vi "X_Y_movePID.vi"() -> ()   [LabVIEW 2023]
doc: "Shows how to move a motor to an absolute position."
panel:
  out "function name out":errorcluster
  out "element 2":dbl
  in  "Home 2":bool
  in  "HWSerialNum 2":i32=83829481
  in  "MG17Motor 2":refnum<k7>(container)
  out "element":dbl
  out "return value":dbl[](array[numeric])
  in  "HWSerialNum":i32=83828425
  in  "MG17Motor":refnum<k7>(container)
  in  "Stop":bool
  in  "Home":bool
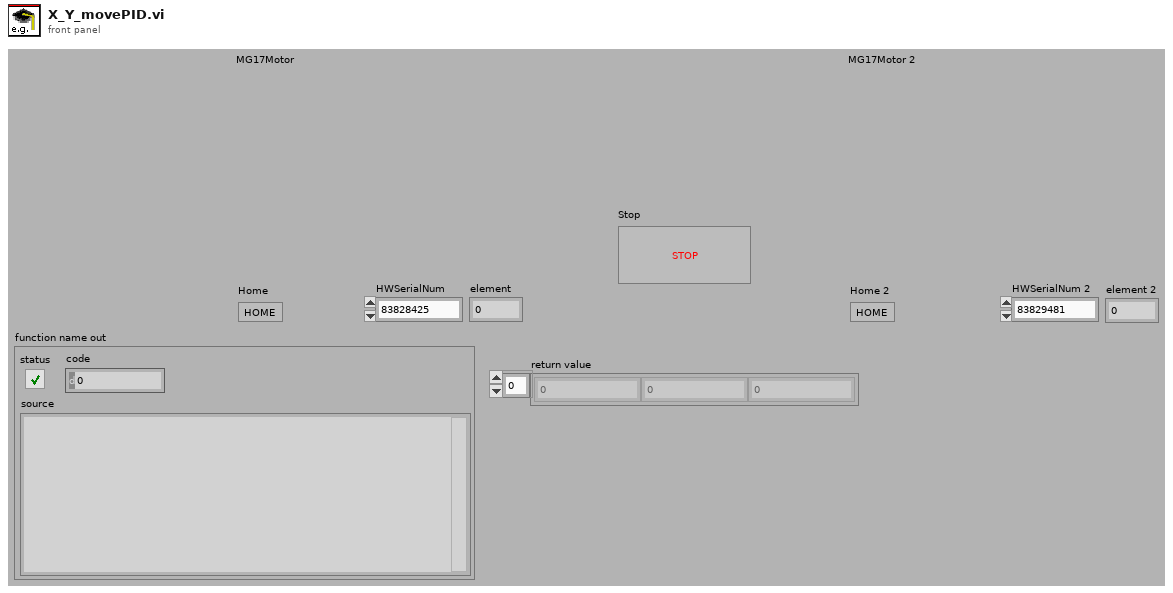
[diagram p1: front panel]
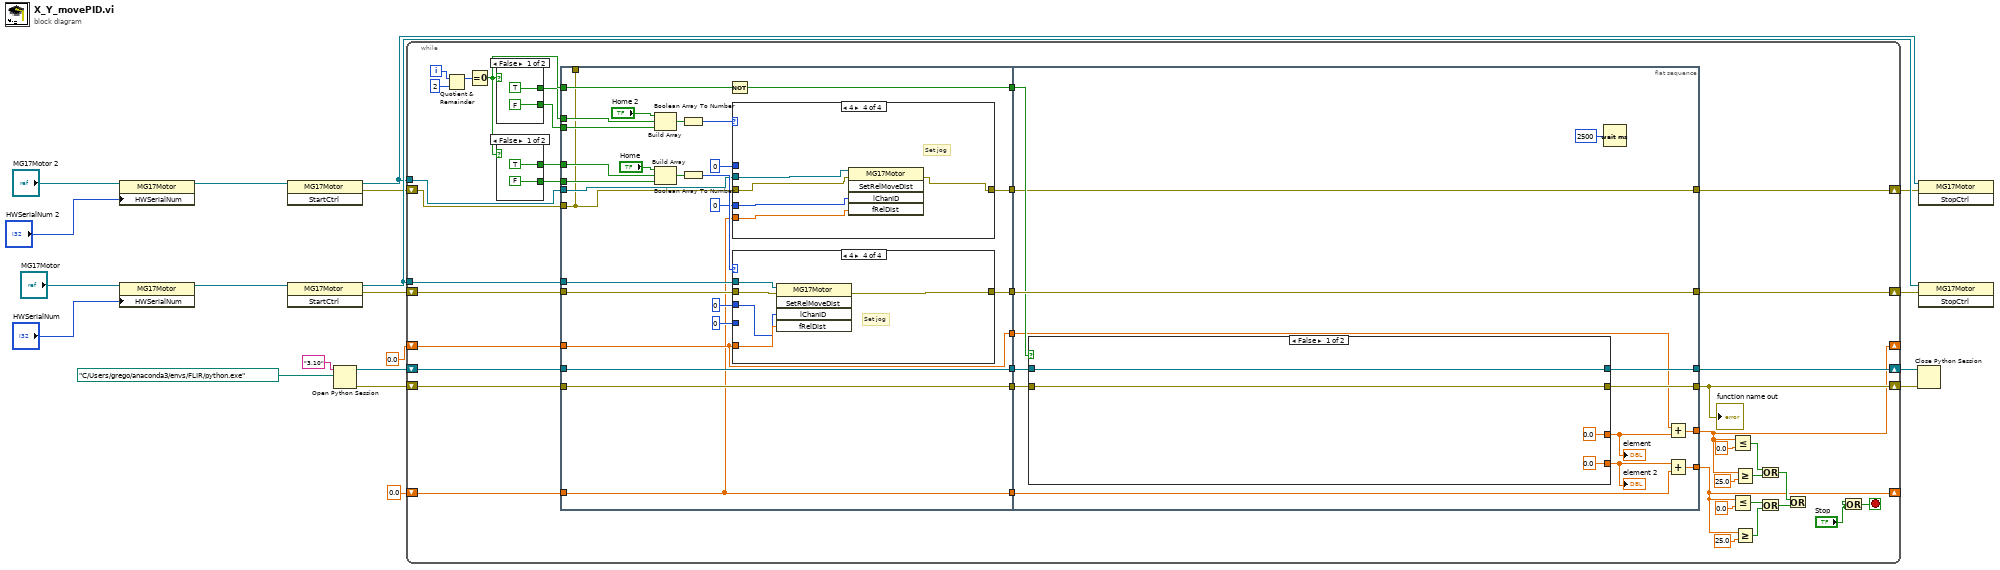
[diagram p0: block diagram]
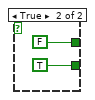
[diagram p2: hidden frame]
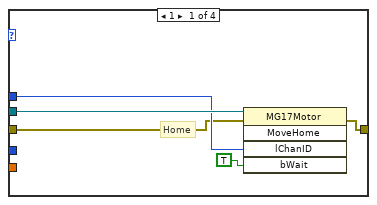
[diagram p3: hidden frame]
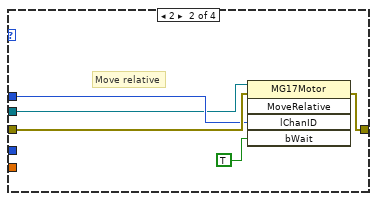
[diagram p4: hidden frame]
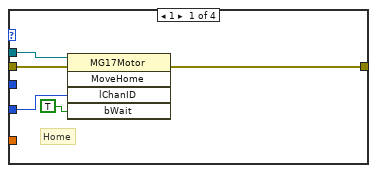
[diagram p6: hidden frame]
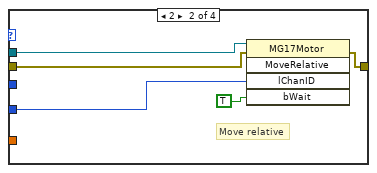
[diagram p7: hidden frame]
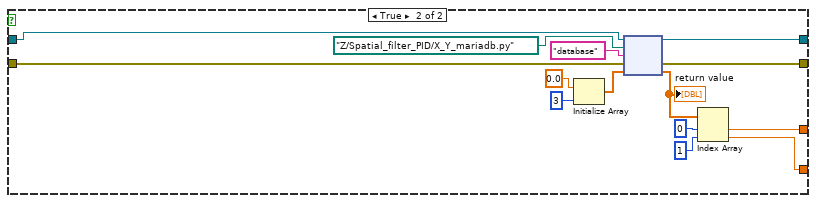
[diagram p9: hidden frame]
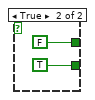
[diagram p10: hidden frame]
diagram:
  n1 = property class="MG17Motor"(reference="MG17Motor 2", "HWSerialNum"="HWSerialNum 2") -> (reference out=w8:refnum<k7>)  [unwired: 1 in, 1 out]
  n2 = property class="MG17Motor"(reference="MG17Motor", "HWSerialNum"="HWSerialNum") -> (reference out=w17:refnum<k7>)  [unwired: 1 in, 1 out]
  n3 = invoke class="MG17Motor" method="StartCtrl"(reference=w8) -> (reference out=w4:refnum<k7>, error out=w3:errorcluster)  [unwired: 2 in, 1 out]
  n4 = invoke class="MG17Motor" method="StartCtrl"(reference=w17) -> (reference out=w20:refnum<k7>, error out=w19:errorcluster)  [unwired: 2 in, 1 out]
  n5 = Open Python Session(python version="3.10" ("Python version"), python path=path "C:/Users/grego/anaconda3/envs/FLIR/python.exe" ("Python path")) -> (session out=w12:refnum<k35>, error out=w11:errorcluster)  [unwired: 1 in]
  n6 = while {
    shift-left: w19 -> [w59]
    shift-right: [w60] -> w18
    tunnel: w20 -> [w61]
    shift-right: [w42] -> _
    shift-left: 0.0 ("p") -> [w53]
    shift-right: [w50] -> w10
    shift-left: w12 -> [w47]
    shift-right: [w49] -> w9
    shift-left: w11 -> [w45]
    tunnel: w4 -> [w36]
    shift-right: [w26] -> _
    shift-left: 0.0 -> [w33]
    shift-right: [w25] -> w5
    shift-left: w3 -> [w23]
    i -> [w57]
    stop <- w24 stop-if-true
    n7 = Quotient & Remainder(x=w57, y=2) -> (x-y*floor(x/y)=w58:i32)  [unwired: 1 out]
    n8 = Equal To 0?(x=w58) -> (x = 0?=w37:bool)
    n9 = case shown="False" w37 {
      tunnel: [TRUE FALSE] -> w35
      tunnel: [FALSE TRUE] -> w34
      frame False {
      }
      frame True {
      }
    }
    n10 = case shown="False" w37 {
      tunnel: [TRUE FALSE] -> w55
      tunnel: [FALSE TRUE] -> w54
      frame False {
      }
      frame True {
      }
    }
    n11 = flat-sequence {
      tunnel: w61 -> [w90]
      tunnel: w59 -> [w87]
      tunnel: w55 -> [w70]
      tunnel: w54 -> [w69]
      tunnel: w53 -> [w79]
      tunnel: w37 -> [w83]
      tunnel: [w88] -> w52
      tunnel: [w82] -> w51
      tunnel: [w81] -> w48
      tunnel: w47 -> [w81]
      tunnel: [w80] -> w46
      tunnel: w45 -> [w80]
      tunnel: [w79] -> w44
      tunnel: w36 -> [w78]
      tunnel: [w66] -> _
      tunnel: w35 -> [w76]
      tunnel: w34 -> [w75]
      tunnel: w33 -> [w67]
      tunnel: [w68] -> w32
      tunnel: [w67] -> w31
      tunnel: w23 -> [w66]
      tunnel: [w137] -> w60
      tunnel: w52 -> [w137]
      tunnel: w51 -> [w134]
      tunnel: [w136] -> w50
      tunnel: [w135] -> w49
      tunnel: [w131] -> w42
      tunnel: w48 -> [w132]
      tunnel: w46 -> [w133]
      tunnel: w44 -> [w130]
      tunnel: w32 -> [w125]
      tunnel: w31 -> [w128]
      tunnel: [w127] -> w26
      tunnel: [w125] -> w25
      frame #0 {
        n12 = Build Array("Home 2", w76, w75) -> (w74:bool[])
        n13 = Build Array("Home", w70, w69) -> (w85:bool[])
        n14 = Boolean Array To Number(Boolean array=w74) -> (number=w73:u32)
        n15 = Boolean Array To Number(Boolean array=w85) -> (number=w86:u32)
        n16 = Not(x=w83) -> (.not. x?=w82:bool)
        n17 = case shown="4" w73 {
          tunnel: w78 -> [w96 w97 _ w105]
          tunnel: 0 ("lChanID") -> [w95 w99 _ _]
          tunnel: w67 -> [_ _ _ w103]
          tunnel: [w94 w101 w102 w107] -> w68
          tunnel: w66 -> [w93 w100 w102 w106]
          tunnel: 0 ("lChanID") -> [_ _ _ w104]
          frame 1 {
            # "Home"
            n18 = invoke class="MG17Motor" method="MoveHome"(reference=w96, error in=w93, "lChanID"=w95, "bWait"=TRUE) -> (error out=w94:errorcluster)  [unwired: 1 in, 4 out]
          }
          frame 2 {
            # "Move relative"
            n19 = invoke class="MG17Motor" method="MoveRelative"(reference=w97, error in=w100, "lChanID"=w99, "bWait"=TRUE) -> (error out=w101:errorcluster)  [unwired: 1 in, 4 out]
          }
          frame Default {
          }
          frame 4 {
            # "Set jog"
            n20 = invoke class="MG17Motor" method="SetRelMoveDist"(reference=w105, error in=w106, "lChanID"=w104, "fRelDist"=w103) -> (error out=w107:errorcluster)  [unwired: 1 in, 4 out]
          }
        }
        n21 = case shown="4" w86 {
          tunnel: w90 -> [w112 w116 _ w119]
          tunnel: 0 ("lChanID") -> [w111 w114 _ _]
          tunnel: w79 -> [_ _ _ w122]
          tunnel: [w110 w117 w118 w123] -> w88
          tunnel: w87 -> [w109 w115 w118 w120]
          tunnel: 0 ("lChanID") -> [_ _ _ w121]
          frame 1 {
            # "Home"
            n22 = invoke class="MG17Motor" method="MoveHome"(reference=w112, error in=w109, "lChanID"=w111, "bWait"=TRUE) -> (error out=w110:errorcluster)  [unwired: 1 in, 4 out]
          }
          frame 2 {
            # "Move relative"
            n23 = invoke class="MG17Motor" method="MoveRelative"(reference=w116, error in=w115, "lChanID"=w114, "bWait"=TRUE) -> (error out=w117:errorcluster)  [unwired: 1 in, 4 out]
          }
          frame Default {
          }
          frame 4 {
            # "Set jog"
            n24 = invoke class="MG17Motor" method="SetRelMoveDist"(reference=w119, error in=w120, "lChanID"=w121, "fRelDist"=w122) -> (error out=w123:errorcluster)  [unwired: 1 in, 4 out]
          }
        }
      }
      frame #1 {
        n25 = case shown="False" w134 {
          tunnel: w132 -> [w141 w145]
          tunnel: w133 -> [w140 w144]
          tunnel: [w141 w150] -> w136
          tunnel: [w140 w149] -> w135
          tunnel: [0.0 w146] -> w129
          tunnel: [0.0 ("element") w142] -> w126
          frame False {
          }
          frame True {
            n26 = Initialize Array(0.0 ("element"), 3 ("dimension size")) -> (w154:dbl[])
            n27 = node(w145, path "Z:/Spatial_filter_PID/X_Y_mariadb.py" ("module path"), "database" ("function name"), w144, w154) -> (w150:refnum<k35>, w149:errorcluster, w148:dbl[])  [unwired: 2 out]
            "return value" <- w148
            n28 = Index Array(array=w148, index #1=0 ("index"), index #2=1 ("index")) -> (element #1=w146:dbl, element #2=w142:dbl)
          }
        }
        "element" <- w129
        "element 2" <- w126
        n29 = Wait (ms)(milliseconds to wait=u32 2500) -> ()  [unwired: 1 out]
        n30 = Add(x=w130, y=w129) -> (x+y=w131:dbl)
        n31 = Add(x=w126, y=w128) -> (x+y=w127:dbl)
      }
    }
    n32 = Less Or Equal?(x=w42, y=0.0) -> (x <= y?=w40:bool)
    n33 = Less Or Equal?(x=w26, y=0.0) -> (x <= y?=w28:bool)
    n34 = Greater Or Equal?(x=w42, y=25.0) -> (x >= y?=w39:bool)
    n35 = Greater Or Equal?(x=w26, y=25.0) -> (x >= y?=w27:bool)
    n36 = Or(x=w40, y=w39) -> (x .or. y?=w38:bool)
    n37 = Or(x=w28, y=w27) -> (x .or. y?=w22:bool)
    n38 = Or(x=w38, y=w22) -> ()  [unwired: 1 out]
    n39 = Or(x="Stop", y="Stop") -> (x .or. y?=w24:bool)
    "function name out" <- w49
  }
  n40 = Close Python Session(session in=w10, error in=w9) -> ()  [unwired: 1 out]
  n41 = invoke class="MG17Motor" method="StopCtrl"(reference=w4, error in=w5) -> ()  [unwired: 1 in, 3 out]
  n42 = invoke class="MG17Motor" method="StopCtrl"(reference=w20, error in=w18) -> ()  [unwired: 1 in, 3 out]
